vi "CFTS-Options Dialog.vi"(0 "Options in":T1, 2 "Parent VI":refnum<vi>) -> (4 "Options out":T1, 10 "Cancelled?":bool=TRUE)   [LabVIEW 2020]
doc: "Use this template to create a dialog box with event handling."
uses:
  epl-vi-lib/Utility VIs/Controls/KBackground Gradient/KBackground Gradient.xctl
  CFTS-Options.ctl
  epl-vi-lib/Utility VIs/Controls/KListboxEx/KListboxEx.xctl
panel:
  in  "Allow nonEPL":bool caption="Allow non-EPL compatible"
  in  "Names":i32(xcontrol)
  in  "Allow all users":bool
  in  "Users":i32(xcontrol)
  in  "Password":bool
  in  "Extension":string caption="Default data file extension"
  in  "Rig name":string
  in  "Help Button":bool
  in  "background":dbl(xcontrol)
  in  "Vitals":bool caption="Auto-start physiological monitor"
  in  "Left":u16(ring) items=["", "ABI-L", "ABI-R", "Left", "Right", "SN24", "SN31", "SN32", "SN36", "SN40", "SN41", "SN42", "Freefield"]
  in  "Right":u16(ring) items=["", "ABI-L", "ABI-R", "Left", "Right", "SN24", "SN31", "SN32", "SN36", "SN40", "SN41", "SN42", "Freefield"]
  in  "Cancel":bool
  in  "OK":bool
  # "Options"
  # "Acoustic System IDs"
  # "Other options"
  # "Advanced users"
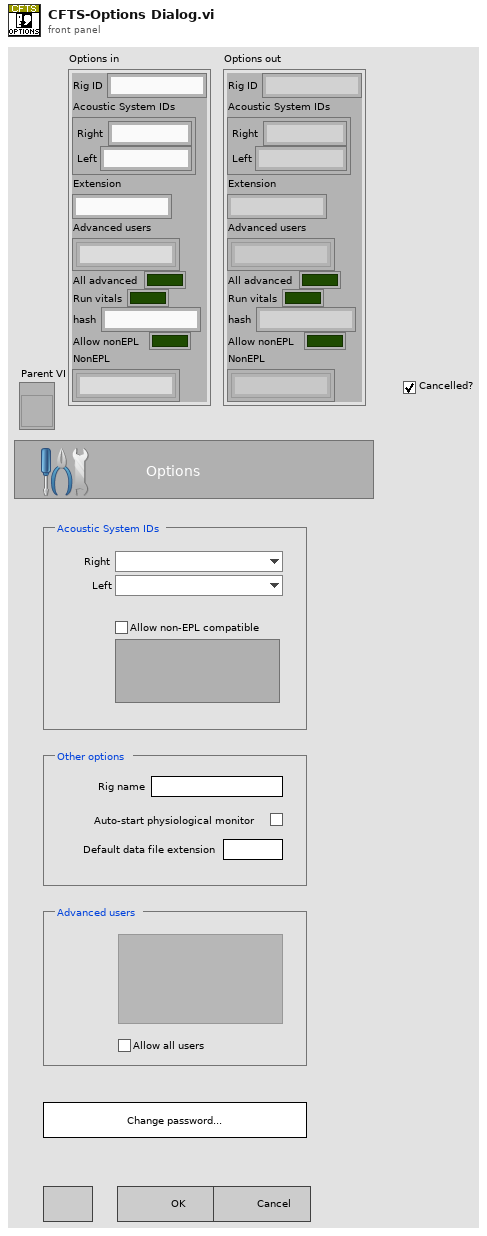
[diagram p1: front panel]
types:
  T1 = typedef "CFTS-Options.ctl" = cluster{"Rig ID":string, "Acoustic System IDs":cluster{"Right":string, "Left":string}, "Extension":string, "Advanced users":string[], "All advanced":bool, "Run vitals":bool, "hash":string, "Allow nonEPL":bool, "NonEPL":string[]}
  T2 = enum8{"Enabled", "Disabled", "Disabled and Grayed Out"}
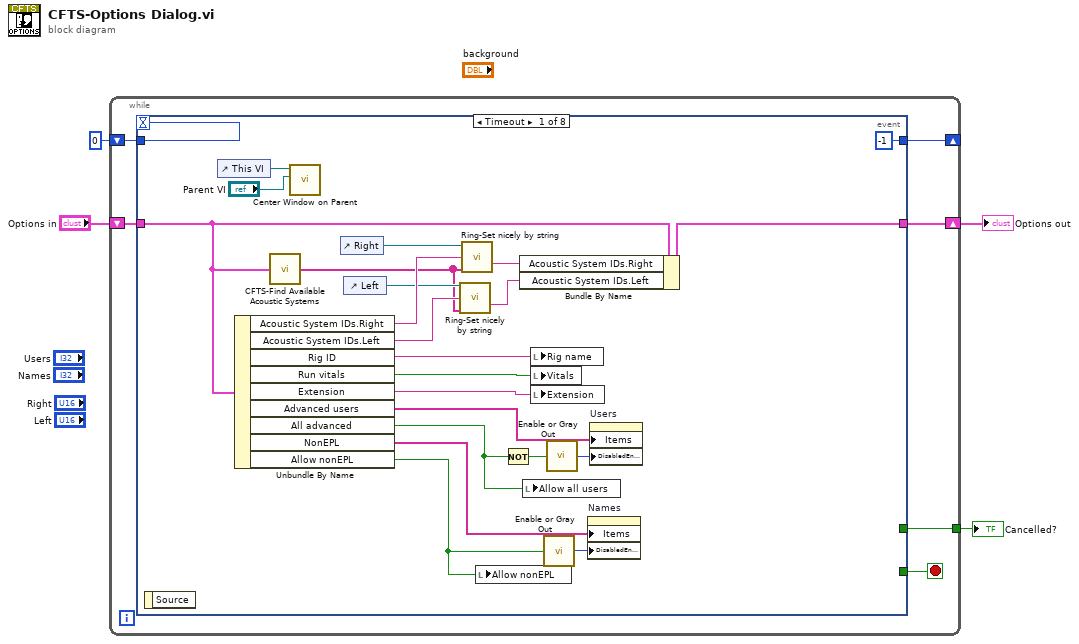
[diagram p0: block diagram]
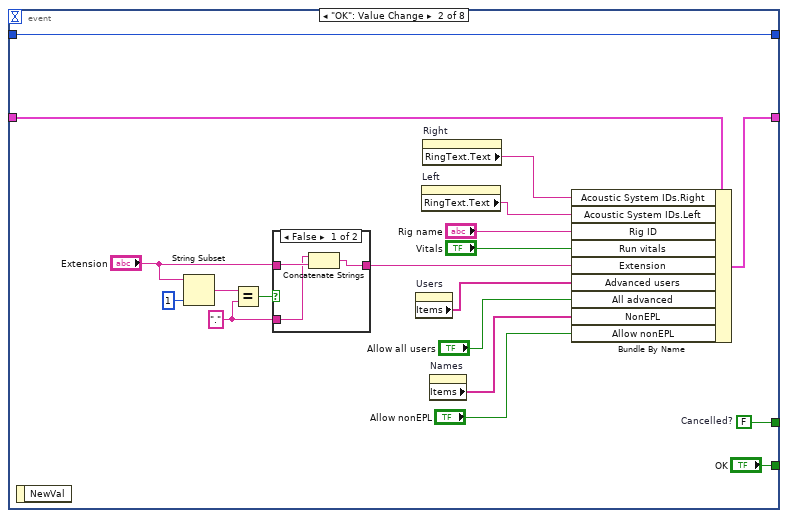
[diagram p2: hidden frame]
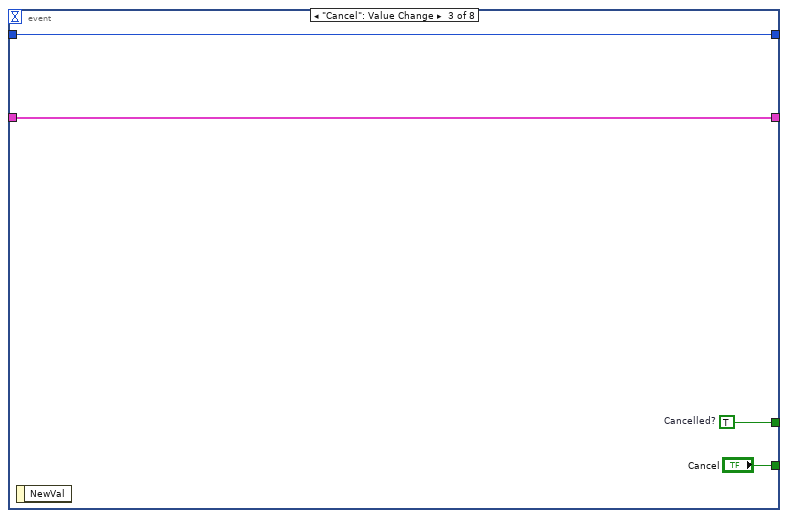
[diagram p4: hidden frame]
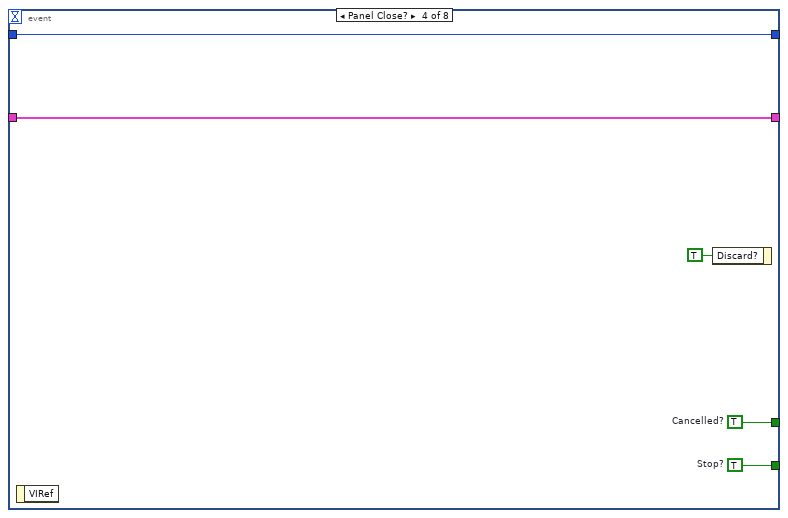
[diagram p5: hidden frame]
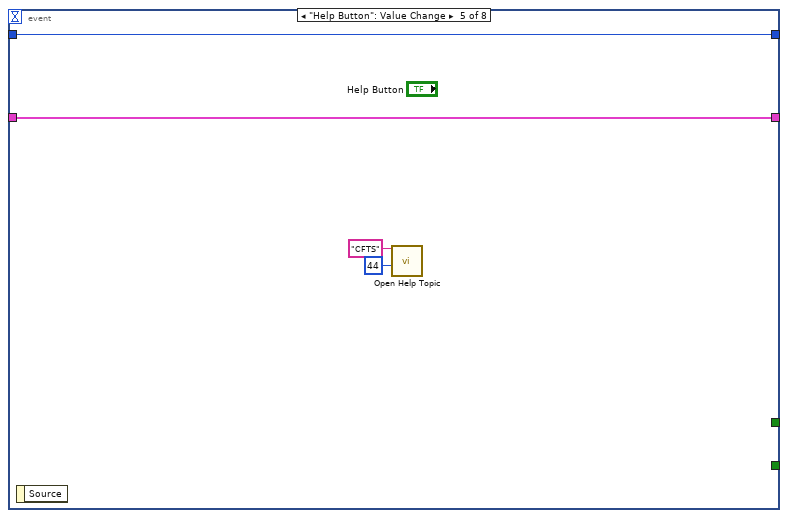
[diagram p6: hidden frame]
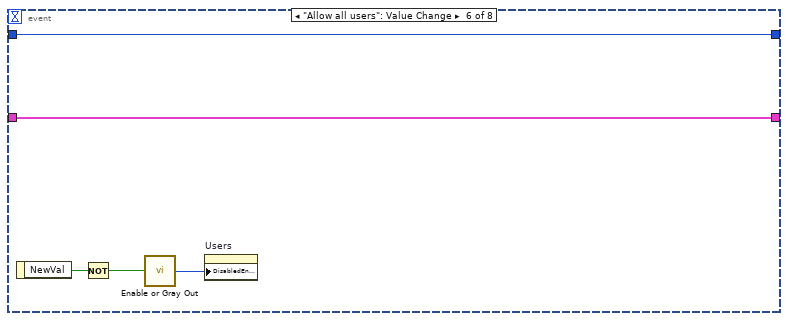
[diagram p7: hidden frame]
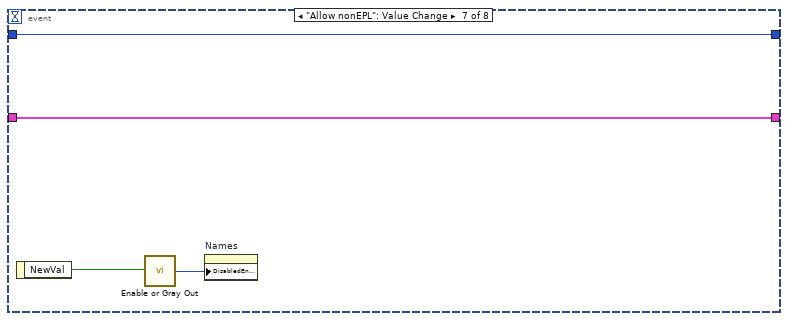
[diagram p8: hidden frame]
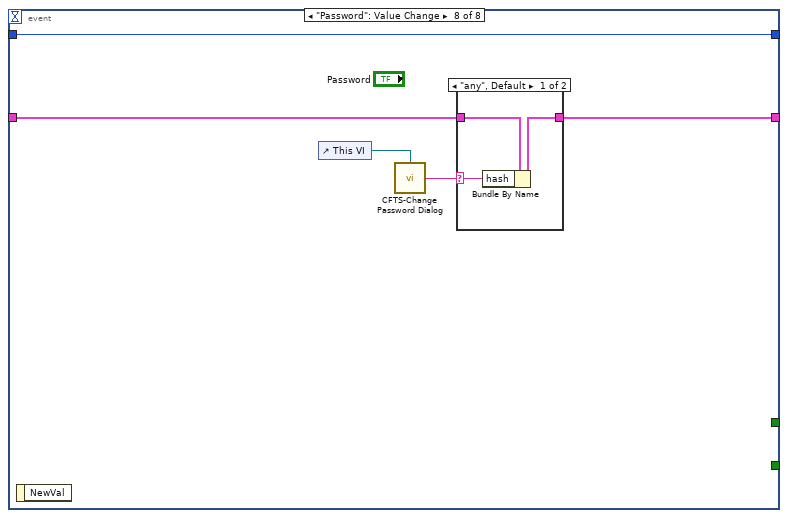
[diagram p9: hidden frame]
diagram:
  n1 = while {
    tunnel: [w9] -> w4
    shift-right: [w8] -> _
    shift-left: 0 -> [w7]
    shift-right: [w6] -> w1
    shift-left: "Options in" -> [w5]
    stop <- w10 stop-if-true
    n2 = event shown="[0] Timeout" {
      selector: _ -> [_ _ _ _ _ _ _ _]
      dyn-events: _ -> [_ _ _ _ _ _ _ _]
      timeout: w7 -> [_ _ _ _ _ _ _ _]
      tunnel: [_ "OK" "Cancel" w63 _ _ _ _] -> w10
      tunnel: [_ w51 w59 w62 _ _ _ _] -> w9
      tunnel: [-1 w48 w57 w61 w68 w73 w77 w82] -> w8
      tunnel: w7 -> [_ w48 w57 w61 w68 w73 w77 w82]
      tunnel: [w15 w41 w56 w60 w67 w72 w76 w78] -> w6
      tunnel: w5 -> [w11 w47 w56 w60 w67 w72 w76 w80]
      event Timeout {
        n3 = event-data() -> ()  [unwired: 1 in, 1 out]
        n4 = control-ref of="This VI"() -> (w28:refnum<vi>)
        n5 = Unbundle By Name(w11) -> ("Acoustic System IDs.Right"=w18:string, "Acoustic System IDs.Left"=w17:string, "Rig ID"=w29:string, "Run vitals"=w31:bool, "Extension"=w30:string, "Advanced users"=w26:string[], "All advanced"=w24:bool, "NonEPL"=w22:string[], "Allow nonEPL"=w20:bool)
        n6 = call "CFTS-Find Available Acoustic Systems.vi"("Options"=w11) -> ("Acoustic Systems"=w12:string[])  [unwired: 14 in]
        n7 = call "Center Window on Parent.vi"("Parent VI"="Parent VI", "VI in"=w28) -> ()  [unwired: 8 in, 2 out]
        n8 = control-ref of="Right"() -> (w19:refnum<vi>)
        n9 = control-ref of="Left"() -> (w16:refnum<vi>)
        n10 = call "Ring-Set nicely by string.vi"("Ring in"=w16, "Device"=w17, "Strings []"=w12) -> ("Selection"=w13:string)  [unwired: 8 in, 4 out]
        n11 = call "Ring-Set nicely by string.vi"("Ring in"=w19, "Device"=w18, "Strings []"=w12) -> ("Selection"=w14:string)  [unwired: 8 in, 4 out]
        n12 = local write "Allow nonEPL"(w20) -> ()
        n13 = Not(x=w24) -> (.not. x?=w23:bool)
        n14 = Bundle By Name(cluster=w11, "Acoustic System IDs.Right"=w14, "Acoustic System IDs.Left"=w13) -> (w15:T1)
        n15 = local write "Allow all users"(w24) -> ()
        n16 = local write "Rig name"(w29) -> ()
        n17 = local write "Vitals"(w31) -> ()
        n18 = local write "Extension"(w30) -> ()
        n19 = call "Enable or Gray Out.vi"("Boolean"=w20) -> ("Disabled"=w21:T2)
        n20 = call "Enable or Gray Out.vi"("Boolean"=w23) -> ("Disabled"=w25:T2)
        n21 = property on="Names" class="KListboxEx (strict)"("Items"=w22, "DisabledEnum"=w21) -> ()  [unwired: 2 in, 2 out]
        n22 = property on="Users" class="KListboxEx (strict)"("Items"=w26, "DisabledEnum"=w25) -> ()  [unwired: 2 in, 2 out]
      }
      event "OK": Value Change {
        w42 = "."
        w51 = FALSE  # Cancelled?
        n23 = event-data() -> ()  [unwired: 1 in, 1 out]
        n24 = String Subset(string="Extension", length (rest)=1 ("length (rest)")) -> (substring=w45:string)  [unwired: 1 in]
        n25 = Equal?(x=w45, y=w42) -> (x = y?=w44:bool)
        n26 = case shown="False" w44 {
          tunnel: "Extension" -> [w54 w55]
          tunnel: w42 -> [w53 _]
          tunnel: [w52 w55] -> w39
          frame False {
            n27 = Concatenate Strings(w53, w54) -> (w52:string)
          }
          frame True {
          }
        }
        n28 = property on="Users" class="KListboxEx (strict)"() -> ("Items"=w38:string[])  [unwired: 2 in, 2 out]
        n29 = property on="Left" class="Ring (strict)"() -> ("RingText.Text"=w33:string)  [unwired: 2 in, 2 out]
        n30 = property on="Right" class="Ring (strict)"() -> ("RingText.Text"=w34:string)  [unwired: 2 in, 2 out]
        n31 = property on="Names" class="KListboxEx (strict)"() -> ("Items"=w36:string[])  [unwired: 2 in, 2 out]
        n32 = Bundle By Name(cluster=w47, "Acoustic System IDs.Right"=w34, "Acoustic System IDs.Left"=w33, "Rig ID"="Rig name", "Run vitals"="Vitals", "Extension"=w39, "Advanced users"=w38, "All advanced"="Allow all users", "NonEPL"=w36, "Allow nonEPL"="Allow nonEPL") -> (w41:T1)
      }
      event "Cancel": Value Change {
        w59 = TRUE  # Cancelled?
        n33 = event-data() -> ()  [unwired: 1 in, 1 out]
      }
      event Panel Close? {
        w62 = TRUE  # Cancelled?
        w63 = TRUE  # Stop?
        n34 = event-data() -> ()  [unwired: 1 in, 1 out]
        n35 = event-data("Discard?"=TRUE) -> ()  [unwired: 1 in, 1 out]
      }
      event "Help Button": Value Change {
        n36 = event-data() -> ()  [unwired: 1 in, 1 out]
        n37 = call "Open Help Topic.vi"("Help file"="CFTS", "HelpId"=44) -> ()  [unwired: 13 in, 1 out]
      }
      event "Allow all users": Value Change {
        n38 = event-data() -> ("NewVal"=w71:bool)  [unwired: 1 in]
        n39 = Not(x=w71) -> (.not. x?=w69:bool)
        n40 = call "Enable or Gray Out.vi"("Boolean"=w69) -> ("Disabled"=w70:T2)
        n41 = property on="Users" class="KListboxEx (strict)"("DisabledEnum"=w70) -> ()  [unwired: 2 in, 2 out]
      }
      event "Allow nonEPL": Value Change {
        n42 = event-data() -> ("NewVal"=w74:bool)  [unwired: 1 in]
        n43 = call "Enable or Gray Out.vi"("Boolean"=w74) -> ("Disabled"=w75:T2)
        n44 = property on="Names" class="KListboxEx (strict)"("DisabledEnum"=w75) -> ()  [unwired: 2 in, 2 out]
      }
      event "Password": Value Change {
        n45 = event-data() -> ()  [unwired: 1 in, 1 out]
        n46 = control-ref of="This VI"() -> (w81:refnum<vi>)
        n47 = call "CFTS-Change Password Dialog.vi"("Parent VI"=w81) -> ("hash"=w79:string)  [unwired: 14 in]
        n48 = case shown="\"any\", Default" w79 {
          selector: w79 -> [w83 _]
          tunnel: w80 -> [w85 w86]
          tunnel: [w84 w86] -> w78
          frame "any", Default {
            n49 = Bundle By Name(cluster=w85, "hash"=w83) -> (w84:T1)
          }
          frame "" {
          }
        }
      }
    }
  }
  "Cancelled?" <- w4
  "Options out" <- w1
